vi "Gen_2D_Raster.vi"(0 "Fast-axis Para":T2={"Number of Steps"=100, "Max X"=5.0, "Min X"=-5.0}, 1 "Lissajous Cluster":cluster{"a":dbl, "b":dbl, "delta":dbl}={"a"=1.0, "b"=2.0, "delta"=0.0} {"delta" format="%_3g"; "b" format="%0.2p"; "a" format="%_3g"}, 2 "error in (no error)":errorcluster, 3 "Soften":bool, 4 "Pattern":T3(ring)=enum."Single Direction (Uniform)", 5 "Reset slow axis at End of Scan?":bool=TRUE, 8 "asymmetry":dbl=0.9, 9 "Soften points":i32=3, 10 "Slow-axis Para":T1={"Number of Steps"=10, "Max Y"=5.0, "Min Y"=-5.0}) -> (6 "2D Raster Pattern":dbl[][](graph)=[[0.0, 0.0, 0.0, 0.0, 0.0, 0.0, 0.0, 0.0, 0.0, 0.0, 0.5555555555555556, 0.5555555555555556, 0.5555555555555556, 0.5555555555555556, 0.5555555555555556, 0.5555555555555556, 0.5555555555555556, 0.5555555555555556, 0.5555555555555556, 0.5555555555555556, 1.1111111111111112, 1.1111111111111112, 1.1111111111111112, 1.1111111111111112, 1.1111111111111112, 1.1111111111111112, 1.1111111111111112, 1.1111111111111112, 1.1111111111111112, 1.1111111111111112, 1.6666666666666667, 1.6666666666666667, 1.6666666666666667, 1.6666666666666667, 1.6666666666666667, 1.6666666666666667, 1.6666666666666667, 1.6666666666666667, 1.6666666666666667, 1.6666666666666667, 2.2222222222222223, 2.2222222222222223, 2.2222222222222223, 2.2222222222222223, 2.2222222222222223, 2.2222222222222223, 2.2222222222222223, 2.2222222222222223, 2.2222222222222223, 2.2222222222222223, 2.7777777777777777, 2.7777777777777777, 2.7777777777777777, 2.7777777777777777, 2.7777777777777777, 2.7777777777777777, 2.7777777777777777, 2.7777777777777777, 2.7777777777777777, 2.7777777777777777, 3.3333333333333335, 3.3333333333333335, 3.3333333333333335, 3.3333333333333335, 3.3333333333333335, 3.3333333333333335, 3.3333333333333335, 3.3333333333333335, 3.3333333333333335, 3.3333333333333335, 3.8888888888888893, 3.8888888888888893, 3.8888888888888893, 3.8888888888888893, 3.8888888888888893, 3.8888888888888893, 3.8888888888888893, 3.8888888888888893, 3.8888888888888893, 3.8888888888888893, 4.444444444444445, 4.444444444444445, 4.444444444444445, 4.444444444444445, 4.444444444444445, 4.444444444444445, 4.444444444444445, 4.444444444444445, 4.444444444444445, 4.444444444444445, 5.0, 5.0, 5.0, 5.0, 5.0, 5.0, 5.0, 5.0, 5.0, 5.0, 5.0, 4.444444444444445, 3.8888888888888893, 3.3333333333333335, 2.7777777777777777, 2.2222222222222223, 1.6666666666666667, 1.1111111111111112, 0.5555555555555556, 0.0], [0.0, 0.5555555555555556, 1.1111111111111112, 1.6666666666666667, 2.2222222222222223, 2.7777777777777777, 3.3333333333333335, 3.8888888888888893, 4.444444444444445, 5.0, 5.0, 4.444444444444445, 3.8888888888888893, 3.3333333333333335, 2.7777777777777777, 2.2222222222222223, 1.6666666666666667, 1.1111111111111112, 0.5555555555555556, 0.0, 0.0, 0.5555555555555556, 1.1111111111111112, 1.6666666666666667, 2.2222222222222223, 2.7777777777777777, 3.3333333333333335, 3.8888888888888893, 4.444444444444445, 5.0, 5.0, 4.444444444444445, 3.8888888888888893, 3.3333333333333335, 2.7777777777777777, 2.2222222222222223, 1.6666666666666667, 1.1111111111111112, 0.5555555555555556, 0.0, 0.0, 0.5555555555555556, 1.1111111111111112, 1.6666666666666667, 2.2222222222222223, 2.7777777777777777, 3.3333333333333335, 3.8888888888888893, 4.444444444444445, 5.0, 5.0, 4.444444444444445, 3.8888888888888893, 3.3333333333333335, 2.7777777777777777, 2.2222222222222223, 1.6666666666666667, 1.1111111111111112, 0.5555555555555556, 0.0, 0.0, 0.5555555555555556, 1.1111111111111112, 1.6666666666666667, 2.2222222222222223, 2.7777777777777777, 3.3333333333333335, 3.8888888888888893, 4.444444444444445, 5.0, 5.0, 4.444444444444445, 3.8888888888888893, 3.3333333333333335, 2.7777777777777777, 2.2222222222222223, 1.6666666666666667, 1.1111111111111112, 0.5555555555555556, 0.0, 0.0, 0.5555555555555556, 1.1111111111111112, 1.6666666666666667, 2.2222222222222223, 2.7777777777777777, 3.3333333333333335, 3.8888888888888893, 4.444444444444445, 5.0, 5.0, 4.444444444444445, 3.8888888888888893, 3.3333333333333335, 2.7777777777777777, 2.2222222222222223, 1.6666666666666667, 1.1111111111111112, 0.5555555555555556, 0.0, 0.0, 0.0, 0.0, 0.0, 0.0, 0.0, 0.0, 0.0, 0.0, 0.0]], 7 "error IO":errorcluster)   [LabVIEW 2014]
uses:
  <vilib>/Analysis/1siggen.llb/Ramp Pattern by Samples.vi
  <vilib>/express/express arith-compare/Formula/XNode/ExpressFormulaBlockNode.xnode
  <vilib>/Analysis/NI_AALBase.lvlib
  <vilib>/gmath/NI_Gmath.lvlib
  <vilib>/measure/NI_MABase.lvlib
panel:
  out "2D  Pattern":dbl[][](graph)
  out "XY Graph 2":cluster{"Y":dbl[], "Y":dbl[]}[](graph) caption="XY Graph"
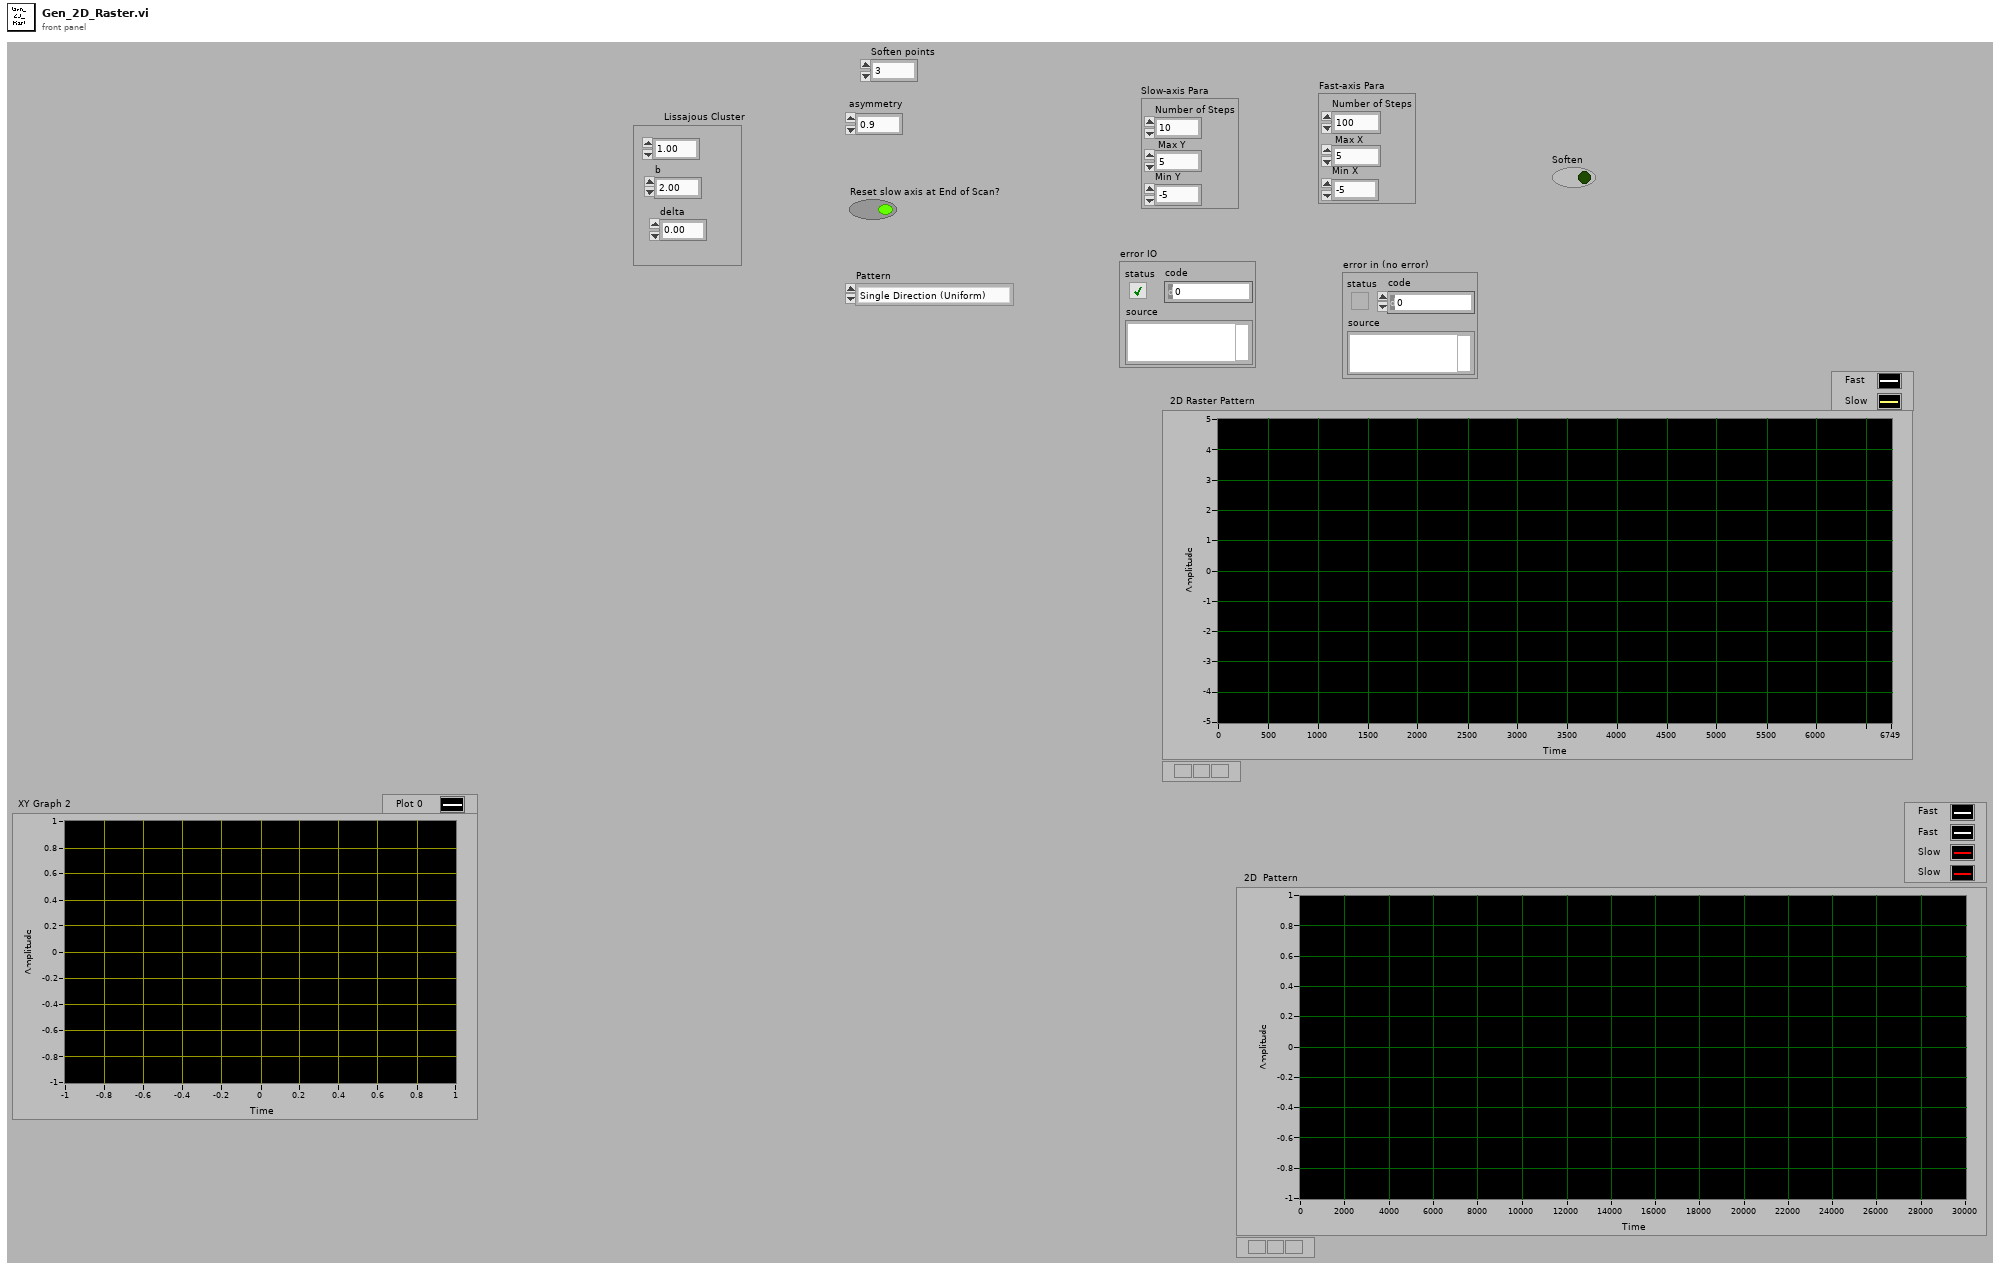
[diagram p1: front panel]
types:
  T1 = cluster{"Number of Steps":i32, "Max Y":dbl, "Min Y":dbl}
  T2 = cluster{"Number of Steps":i32, "Max X":dbl, "Min X":dbl}
  T3 = enum16{"Lissajous", "Adjustable sawtooth", "Single Direction (Uniform)", "Single Direction (Fast Reset)", "Bi-Directional"}
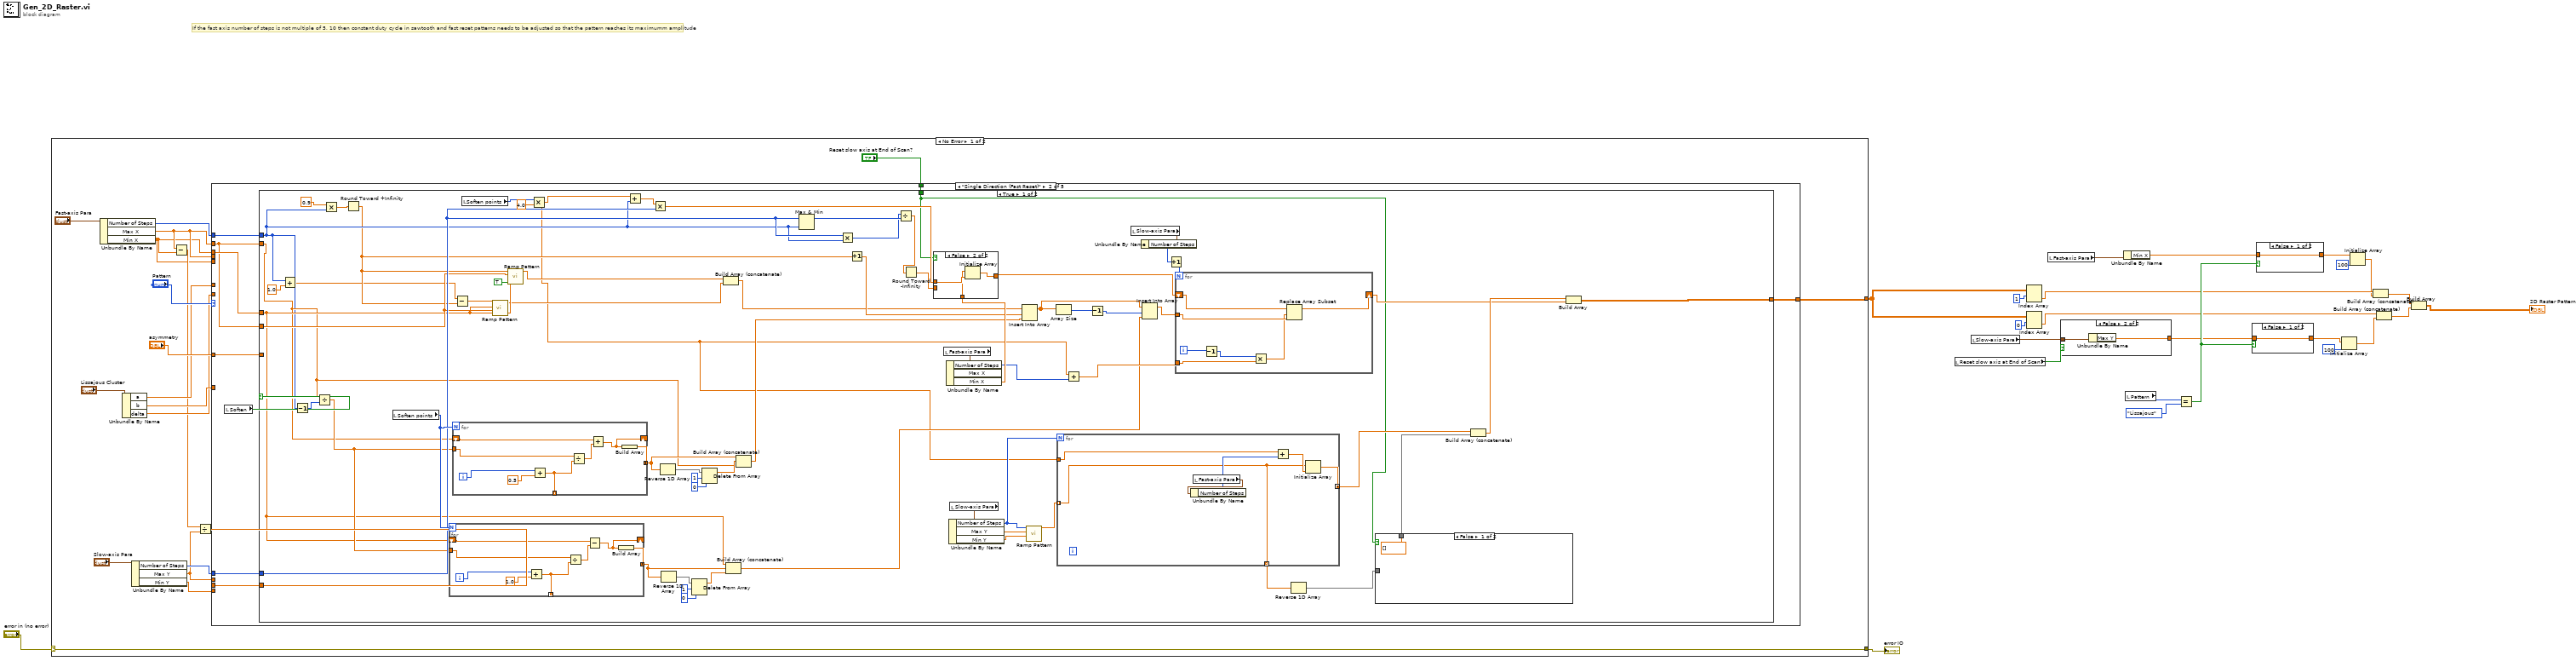
[diagram p0: block diagram]
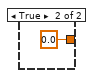
[diagram p2: hidden frame]
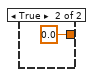
[diagram p3: hidden frame]
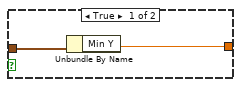
[diagram p4: hidden frame]
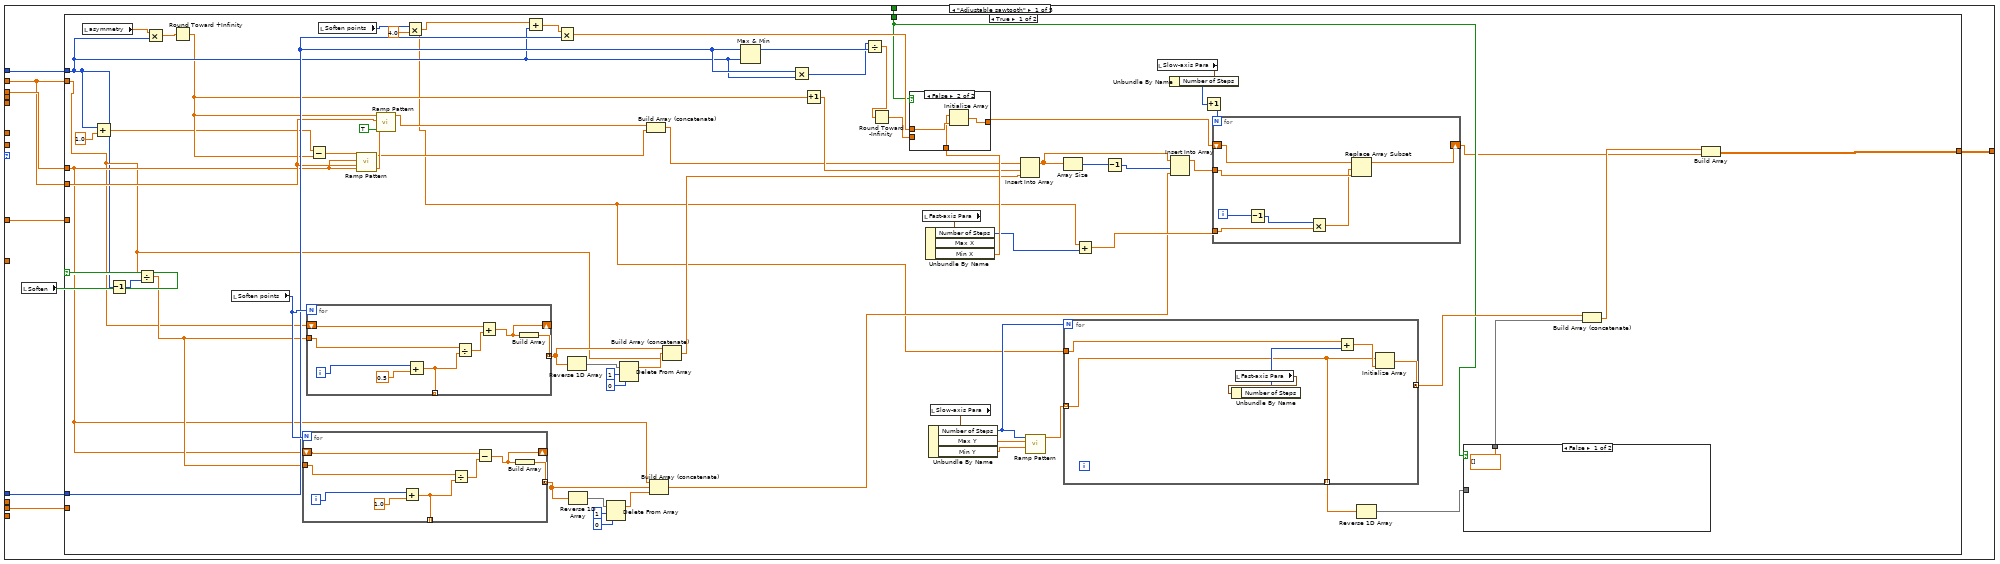
[diagram p5: hidden frame]
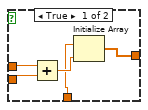
[diagram p7: hidden frame]
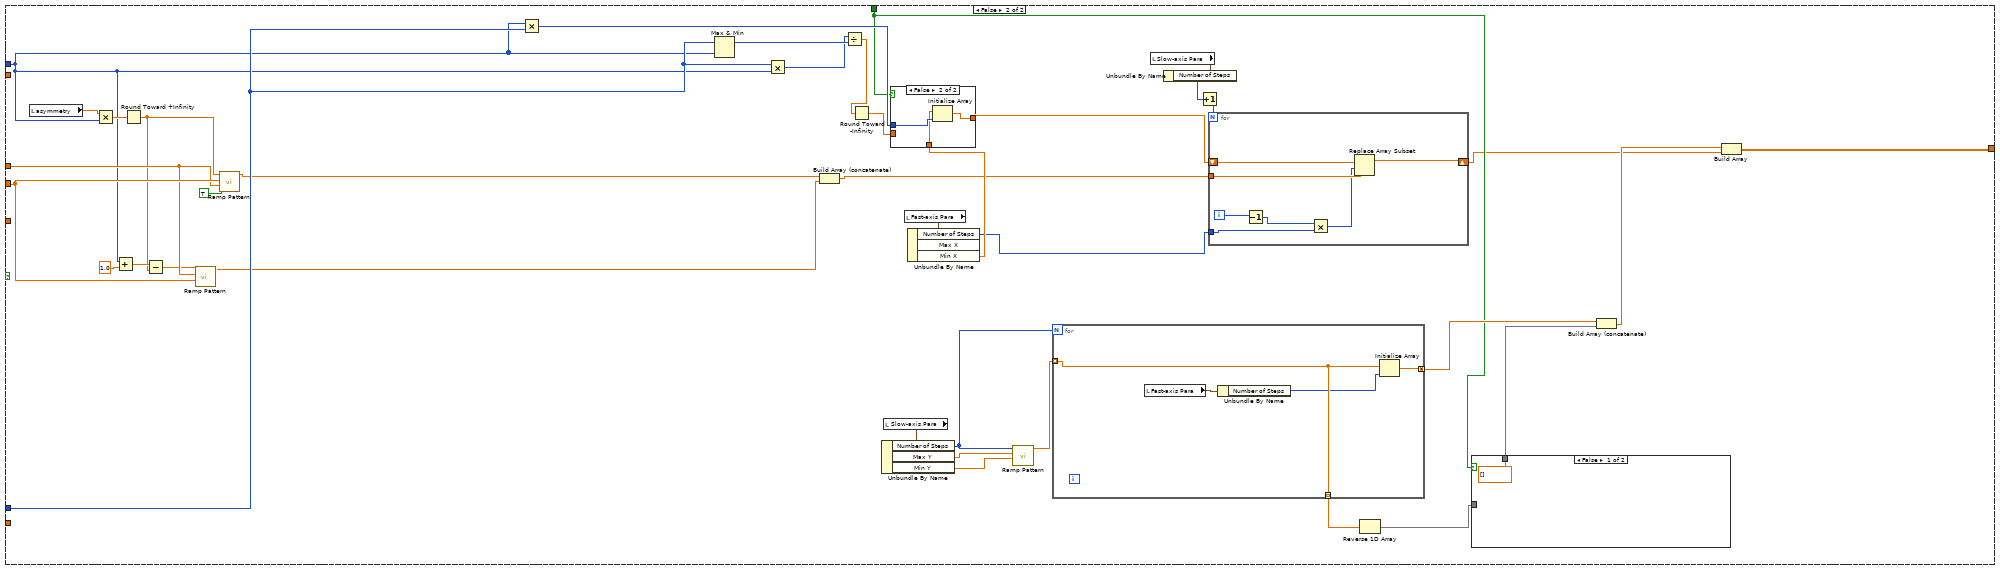
[diagram p8: hidden frame]
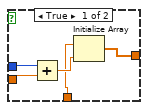
[diagram p10: hidden frame]
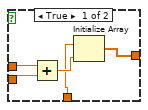
[diagram p12: hidden frame]
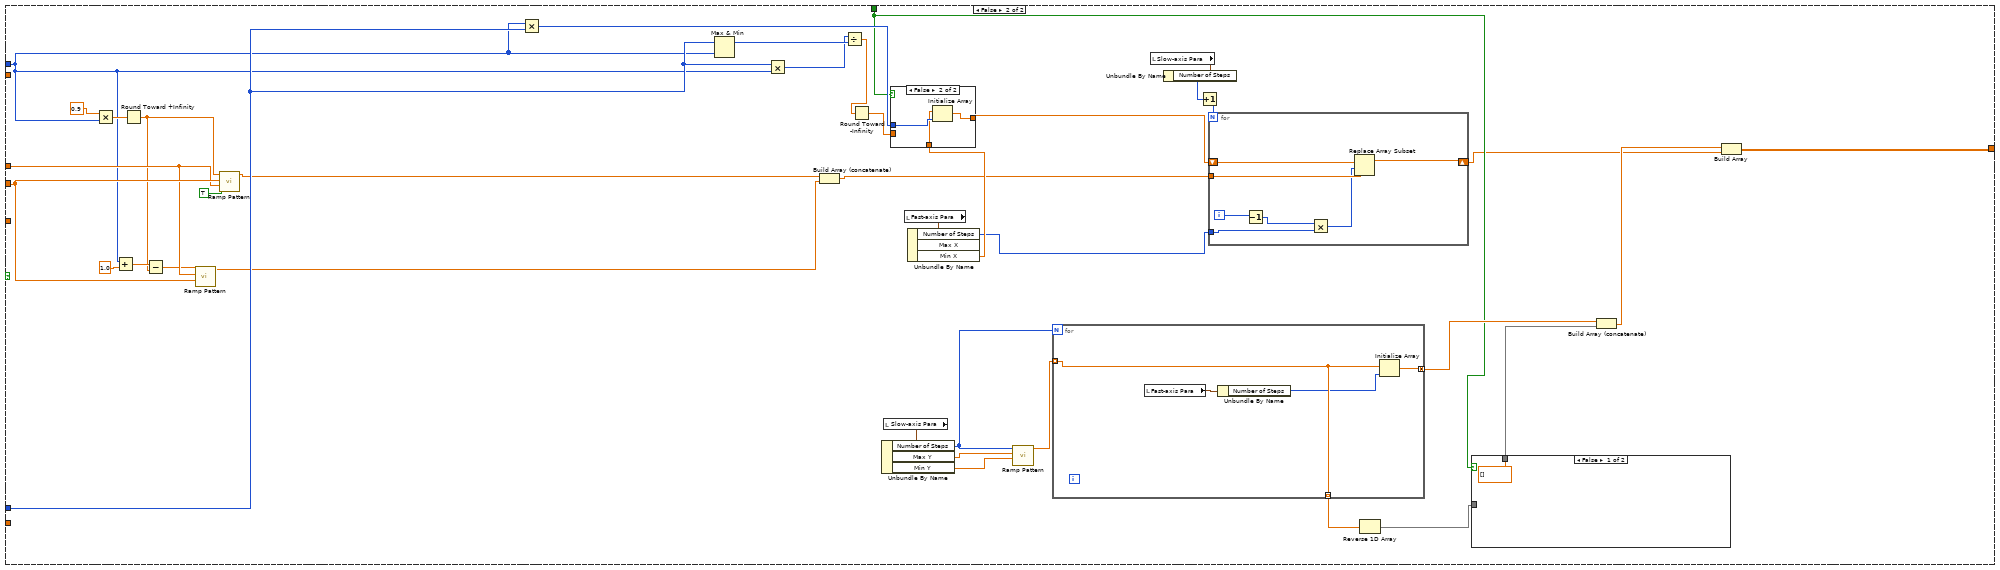
[diagram p13: hidden frame]
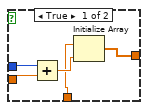
[diagram p15: hidden frame]
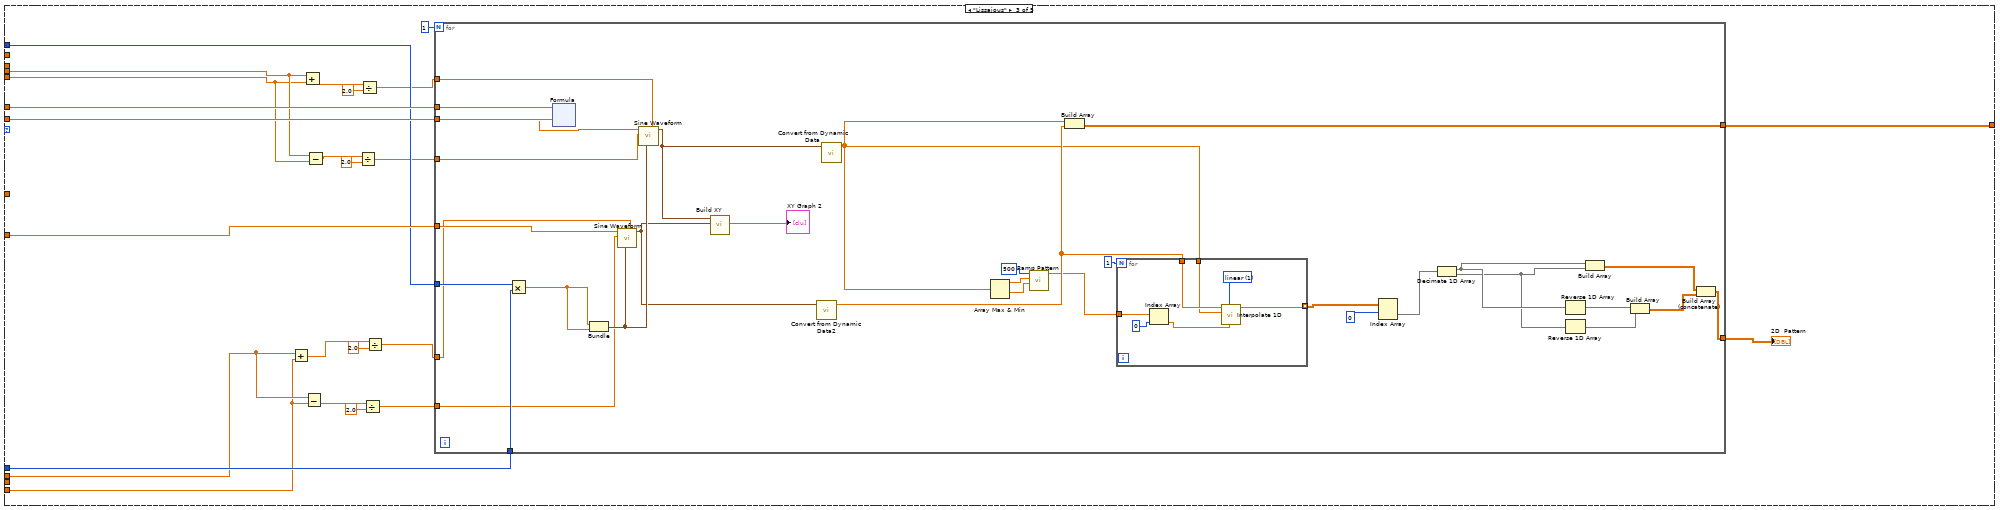
[diagram p16: hidden frame]
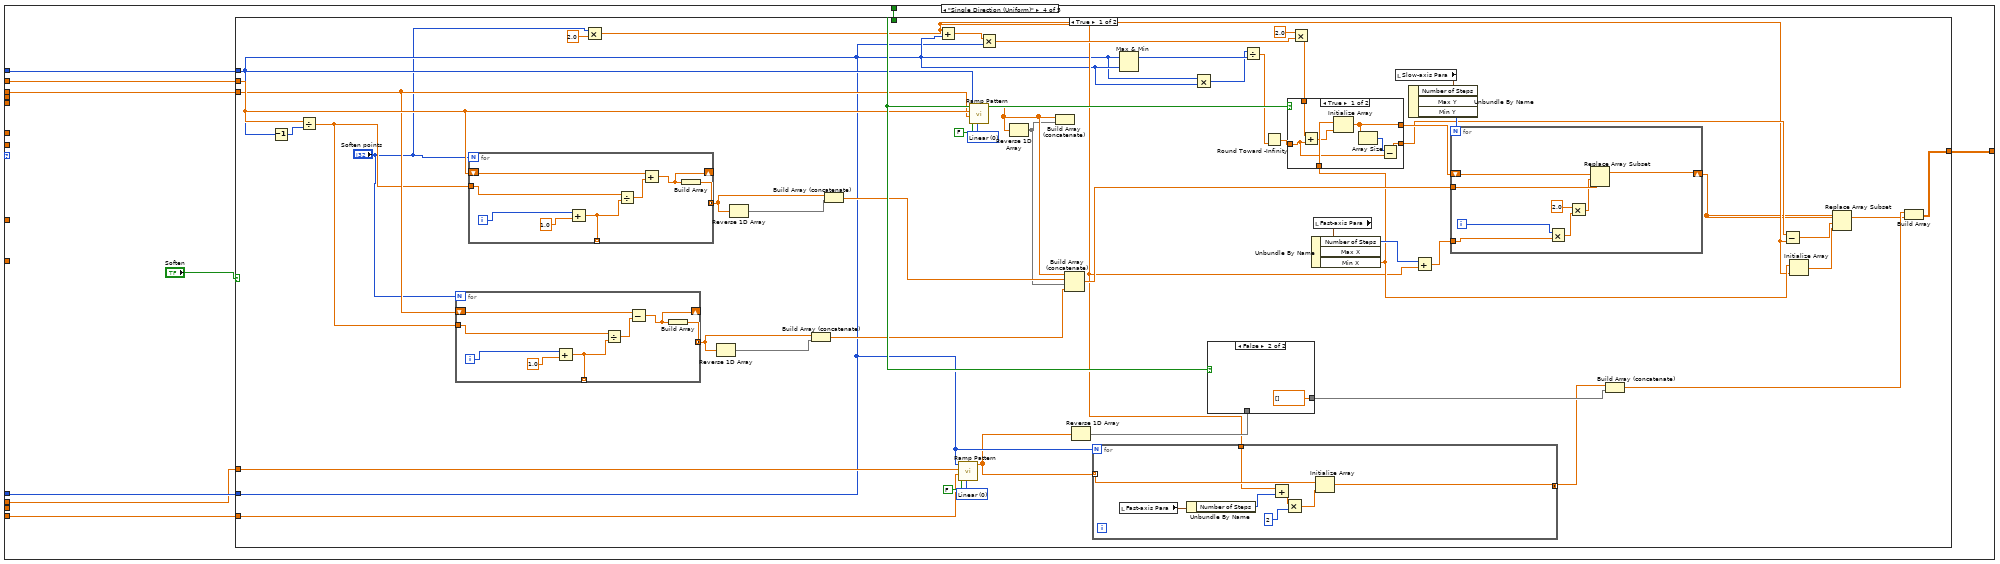
[diagram p17: hidden frame]
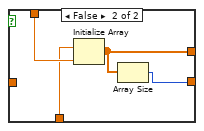
[diagram p19: hidden frame]
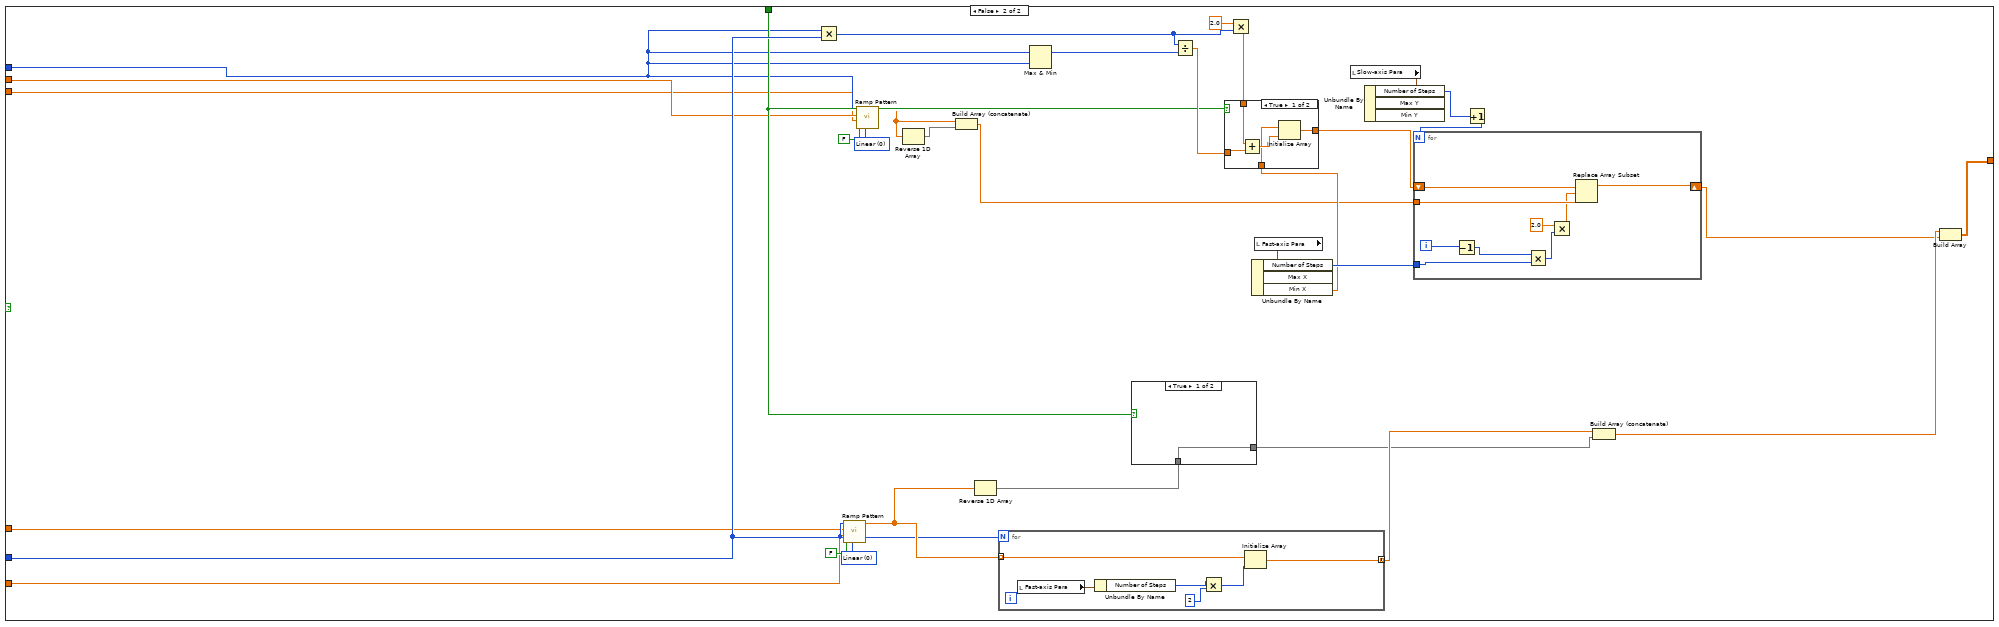
[diagram p20: hidden frame]
diagram:
  # "If the fast axis number of steps is not multiple of 5, 10 then constant duty cycle in sawtooth and fast reset patterns needs to be adjusted so that the pattern reaches its maximumm amplitude"
  n1 = case shown="No Error" "error in (no error)" {
    selector: "error in (no error)" -> [w38 w825]
    tunnel: [w38 w825] -> w21
    tunnel: [w25 dbl[][] []] -> w24
    frame No Error {
      n2 = Unbundle By Name("Fast-axis Para") -> ("Number of Steps"=w41:i32, "Max X"=w27:dbl, "Min X"=w26:dbl)
      n3 = Unbundle By Name("Lissajous Cluster") -> ("a"=w33:dbl, "b"=w34:dbl, "delta"=w32:dbl)
      n4 = Unbundle By Name("Slow-axis Para") -> ("Number of Steps"=w39:i32, "Max Y"=w31:dbl, "Min Y"=w28:dbl)
      n5 = Subtract(x=w27, y=w26) -> (x-y=w29:dbl)
      n6 = Divide(x=w29, y=w31) -> (x/y=w30:dbl)
      n7 = case shown="\"Single Direction (Fast Reset)\"" "Pattern" {
        tunnel: w41 -> [w49 w222 w410 w467 w634]
        tunnel: w27 -> [w44 w217 _ w466 w632]
        tunnel: w26 -> [w52 w225 _ w465 w631]
        tunnel: w30 -> [w51 w224 _ _ _]
        tunnel: w39 -> [w50 w223 w409 w472 w627]
        tunnel: "asymmetry" -> [w47 w220 _ _ _]
        tunnel: [w48 w221 w406 w470 w628] -> w25
        tunnel: "Reset slow axis at End of Scan?" -> [w46 w219 _ w471 w633]
        tunnel: w33 -> [_ _ w413 _ _]
        tunnel: w32 -> [_ _ w412 _ _]
        tunnel: w34 -> [_ _ w411 _ _]
        tunnel: w31 -> [_ _ w394 w469 w630]
        tunnel: w28 -> [_ _ w393 w468 w629]
        tunnel: w27 -> [_ _ w405 _ _]
        tunnel: w26 -> [_ _ w404 _ _]
        frame "Adjustable sawtooth" {
          n8 = local read "Soften"() -> (w45:bool)
          n9 = case shown="True" w45 {
            tunnel: w44 -> [w71 _]
            tunnel: w52 -> [w75 w173]
            tunnel: w51 -> [_ _]
            tunnel: w50 -> [w79 w176]
            tunnel: w49 -> [w69 w157]
            tunnel: [w111 w189] -> w48
            tunnel: w47 -> [_ _]
            tunnel: w46 -> [w82 w179]
            tunnel: w44 -> [w76 w174]
            frame True {
              n10 = local read "asymmetry"() -> (w74:dbl)
              n11 = Add(x=w69, y=1.0) -> (x+y=w59:dbl)
              n12 = Decrement(x=w69) -> (x-1=w99:i32)
              n13 = Divide(x=w71, y=w99) -> (x/y=w77:dbl)
              n14 = Multiply(x=w74, y=w69) -> (x*y=w73:dbl)
              n15 = Round Toward +Infinity(x=w73) -> (ceil(x): smallest int >= x=w60:dbl)
              n16 = local read "Soften points"() -> (w93:i32)
              n17 = for {
                N: w93 -> [_]
                tunnel: w77 -> [w123]
                tunnel: [w124] -> w98 mode=concatenating
                shift-right: [w121] -> _
                shift-left: w75 -> [w125]
                tunnel: [w118] -> _ mode=indexing
                i -> [w119]
                n18 = Add(x=w119, y=1.0) -> (x+y=w118:dbl)
                n19 = Divide(x=w123, y=w118) -> (x/y=w120:dbl)
                n20 = Subtract(x=w125, y=w120) -> (x-y=w121:dbl)
                n21 = Build Array(w121) -> (w124:dbl[])
              }
              n22 = for {
                N: w93 -> [_]
                tunnel: w77 -> [w131]
                tunnel: [w132] -> w103 mode=concatenating
                shift-right: [w129] -> _
                shift-left: w71 -> [w133]
                tunnel: [w126] -> _ mode=indexing
                i -> [w127]
                n23 = Add(x=w127, y=0.5) -> (x+y=w126:dbl)
                n24 = Divide(x=w131, y=w126) -> (x/y=w128:dbl)
                n25 = Add(x=w133, y=w128) -> (x+y=w129:dbl)
                n26 = Build Array(w129) -> (w132:dbl[])
              }
              n27 = Subtract(x=w59, y=w60) -> (x-y=w70:dbl)
              n28 = local read "Soften points"() -> (w88:i32)
              n29 = call-poly <vilib>:"Ramp Pattern.vi"("start"=w76, "end"=w75, "samples"=w70) -> ("Ramp Pattern"=w56:dbl[])  [unwired: 7 in, 1 out]
              n30 = call-poly <vilib>:"Ramp Pattern.vi"("exclude end?"=TRUE, "start"=w75, "end"=w76, "samples"=w60) -> ("Ramp Pattern"=w58:dbl[])  [unwired: 6 in, 1 out]
              n31 = Multiply(x=w88, y=4.0) -> (x*y=w54:dbl)
              n32 = Add(x=w54, y=w69) -> (x+y=w87:dbl)
              n33 = Multiply(x=w87, y=w79) -> (x*y=w116:dbl)
              n34 = Reverse 1D Array(array=w103) -> (reversed array=w102:dbl[])
              n35 = Reverse 1D Array(array=w98) -> (reversed array=w97:dbl[])
              n36 = Delete From Array(array=w97, length=1, index=0) -> (array with subset deleted=w94:dbl[])  [unwired: 1 out]
              n37 = Delete From Array(array=w102, length=1, index=0) -> (array with subset deleted=w91:dbl[])  [unwired: 1 out]
              n38 = Build Array (concatenate)(w58, w56) -> (w67:dbl[])
              n39 = Build Array (concatenate)(w75, w98, w94) -> (w55:dbl[])
              n40 = Build Array (concatenate)(w103, w91, w71) -> (w57:dbl[])
              n41 = Max & Min(x=w79, y=w69) -> (max(x,y)=w115:i32)  [unwired: 1 out]
              n42 = Multiply(x=w79, y=w69) -> (x*y=w78:i32)
              n43 = Increment(x=w60) -> (x+1=w92:dbl)
              n44 = Divide(x=w78, y=w115) -> (x/y=w86:dbl)
              n45 = Round Toward -Infinity(1:w86) -> (0:w85:dbl)
              n46 = local read "Fast-axis Para"() -> (w114:T2)
              n47 = Unbundle By Name(w114) -> ("Number of Steps"=w84:i32, "Min X"=w108:dbl)  [unwired: 1 out]
              n48 = case shown="False" w82 {
                tunnel: [w140 w143] -> w117
                tunnel: w116 -> [w139 w142]
                tunnel: w85 -> [w138 _]
                tunnel: w108 -> [w136 w141]
                frame True {
                  n49 = Add(x=w139, y=w138) -> (x+y=w137:dbl)
                  n50 = Initialize Array(w136, w137) -> (w140:dbl[])
                }
                frame False {
                  n51 = Initialize Array(w141, w142) -> (w143:dbl[])
                }
              }
              n52 = local read "Slow-axis Para"() -> (w112:T1)
              n53 = Unbundle By Name(w112) -> ("Number of Steps"=w64:i32, "Max Y"=w63:dbl, "Min Y"=w62:dbl)
              n54 = Insert Into Array(array=w67, index=w92, new element=w57) -> (w90:dbl[])
              n55 = call-poly <vilib>:"Ramp Pattern.vi"("start"=w62, "end"=w63, "samples"=w64) -> ("Ramp Pattern"=w61:dbl[])  [unwired: 7 in, 1 out]
              n56 = Array Size(array=w90) -> (size(s)=w66:i32)
              n57 = for {
                N: w64 -> [_]
                tunnel: w61 -> [w144] mode=indexing
                tunnel: [w148] -> w104 mode=concatenating
                tunnel: [w144] -> w106 mode=indexing
                tunnel: w54 -> [w147]
                n58 = local read "Fast-axis Para"() -> (w149:T2)
                n59 = Unbundle By Name(w149) -> ("Number of Steps"=w146:i32)
                n60 = Add(x=w147, y=w146) -> (x+y=w145:dbl)
                n61 = Initialize Array(w144, w145) -> (w148:dbl[])
              }
              n62 = Add(x=w54, y=w84) -> (x+y=w83:dbl)
              n63 = Decrement(x=w66) -> (x-1=w65:i32)
              n64 = local read "Slow-axis Para"() -> (w113:T1)
              n65 = Unbundle By Name(w113) -> ("Number of Steps"=w110:i32)
              n66 = Insert Into Array(array=w90, index=w65, new element=w55) -> (w53:dbl[])
              n67 = Increment(x=w110) -> (x+1=w109:i32)
              n68 = for {
                N: w109 -> [_]
                tunnel: w53 -> [w156]
                shift-right: [w154] -> w80
                shift-left: w117 -> [w155]
                tunnel: w83 -> [w152]
                i -> [w151]
                n69 = Decrement(x=w151) -> (x-1=w150:i32)
                n70 = Multiply(x=w150, y=w152) -> (x*y=w153:dbl)
                n71 = Replace Array Subset(array=w155, new element=w156, index=w153) -> (w154:dbl[])
              }
              n72 = Reverse 1D Array(array=w106) -> (reversed array=w105:dbl[])
              n73 = case shown="False" w82 {
                tunnel: w105 -> [_ w135]
                tunnel: [dbl[] [] w135] -> w107
                frame False {
                }
                frame True {
                }
              }
              n74 = Build Array (concatenate)(w104, w107) -> (w81:dbl[])
              n75 = Build Array(w81, w80) -> (w111:dbl[][])
            }
            frame False {
              n76 = local read "asymmetry"() -> (w172:dbl)
              n77 = Multiply(x=w172, y=w157) -> (x*y=w171:dbl)
              n78 = Add(x=w157, y=1.0) -> (x+y=w169:dbl)
              n79 = Round Toward +Infinity(x=w171) -> (ceil(x): smallest int >= x=w160:dbl)
              n80 = Subtract(x=w169, y=w160) -> (x-y=w168:dbl)
              n81 = call-poly <vilib>:"Ramp Pattern.vi"("start"=w174, "end"=w173, "samples"=w168) -> ("Ramp Pattern"=w166:dbl[])  [unwired: 7 in, 1 out]
              n82 = call-poly <vilib>:"Ramp Pattern.vi"("exclude end?"=TRUE, "start"=w173, "end"=w174, "samples"=w160) -> ("Ramp Pattern"=w165:dbl[])  [unwired: 6 in, 1 out]
              n83 = Multiply(x=w157, y=w176) -> (x*y=w194:i32)
              n84 = Max & Min(x=w176, y=w157) -> (max(x,y)=w193:i32)  [unwired: 1 out]
              n85 = Multiply(x=w176, y=w157) -> (x*y=w175:i32)
              n86 = Build Array (concatenate)(w165, w166) -> (w159:dbl[])
              n87 = Divide(x=w175, y=w193) -> (x/y=w181:dbl)
              n88 = Round Toward -Infinity(1:w181) -> (0:w180:dbl)
              n89 = local read "Slow-axis Para"() -> (w190:T1)
              n90 = Unbundle By Name(w190) -> ("Number of Steps"=w164:i32, "Max Y"=w163:dbl, "Min Y"=w162:dbl)
              n91 = local read "Fast-axis Para"() -> (w192:T2)
              n92 = Unbundle By Name(w192) -> ("Number of Steps"=w158:i32, "Min X"=w186:dbl)  [unwired: 1 out]
              n93 = case shown="False" w179 {
                tunnel: [w202 w205] -> w195
                tunnel: w194 -> [w201 w204]
                tunnel: w180 -> [w200 _]
                tunnel: w186 -> [w198 w203]
                frame True {
                  n94 = Add(x=w201, y=w200) -> (x+y=w199:dbl)
                  n95 = Initialize Array(w198, w199) -> (w202:dbl[])
                }
                frame False {
                  n96 = Initialize Array(w203, w204) -> (w205:dbl[])
                }
              }
              n97 = call-poly <vilib>:"Ramp Pattern.vi"("start"=w162, "end"=w163, "samples"=w164) -> ("Ramp Pattern"=w161:dbl[])  [unwired: 7 in, 1 out]
              n98 = for {
                N: w164 -> [_]
                tunnel: w161 -> [w207] mode=indexing
                tunnel: [w208] -> w182 mode=concatenating
                tunnel: [w207] -> w184 mode=indexing
                n99 = local read "Fast-axis Para"() -> (w209:T2)
                n100 = Unbundle By Name(w209) -> ("Number of Steps"=w206:i32)
                n101 = Initialize Array(w207, w206) -> (w208:dbl[])
              }
              n102 = local read "Slow-axis Para"() -> (w191:T1)
              n103 = Unbundle By Name(w191) -> ("Number of Steps"=w188:i32)
              n104 = Increment(x=w188) -> (x+1=w187:i32)
              n105 = for {
                N: w187 -> [_]
                tunnel: w159 -> [w216]
                shift-right: [w214] -> w177
                shift-left: w195 -> [w215]
                tunnel: w158 -> [w212]
                i -> [w211]
                n106 = Decrement(x=w211) -> (x-1=w210:i32)
                n107 = Multiply(x=w210, y=w212) -> (x*y=w213:i32)
                n108 = Replace Array Subset(array=w215, new element=w216, index=w213) -> (w214:dbl[])
              }
              n109 = Reverse 1D Array(array=w184) -> (reversed array=w183:dbl[])
              n110 = case shown="False" w179 {
                tunnel: w183 -> [_ w197]
                tunnel: [dbl[] [] w197] -> w185
                frame False {
                }
                frame True {
                }
              }
              n111 = Build Array (concatenate)(w182, w185) -> (w178:dbl[])
              n112 = Build Array(w178, w177) -> (w189:dbl[][])
            }
          }
        }
        frame "Single Direction (Fast Reset)" {
          n113 = local read "Soften"() -> (w218:bool)
          n114 = case shown="True" w218 {
            tunnel: w217 -> [w246 _]
            tunnel: w225 -> [w249 w346]
            tunnel: w224 -> [_ _]
            tunnel: w223 -> [w253 w349]
            tunnel: w222 -> [w244 w331]
            tunnel: [w284 w362] -> w221
            tunnel: w220 -> [_ _]
            tunnel: w219 -> [w226 w352]
            tunnel: w217 -> [w250 w347]
            frame True {
              n115 = Add(x=w244, y=1.0) -> (x+y=w234:dbl)
              n116 = Decrement(x=w244) -> (x-1=w272:i32)
              n117 = Divide(x=w246, y=w272) -> (x/y=w251:dbl)
              n118 = Multiply(x=0.9 ("asymmetry"), y=w244) -> (x*y=w248:dbl)
              n119 = Round Toward +Infinity(x=w248) -> (ceil(x): smallest int >= x=w235:dbl)
              n120 = local read "Soften points"() -> (w266:i32)
              n121 = for {
                N: w266 -> [_]
                tunnel: w251 -> [w296]
                tunnel: [w297] -> w271 mode=concatenating
                shift-right: [w294] -> _
                shift-left: w249 -> [w298]
                tunnel: [w291] -> _ mode=indexing
                i -> [w292]
                n122 = Add(x=w292, y=1.0) -> (x+y=w291:dbl)
                n123 = Divide(x=w296, y=w291) -> (x/y=w293:dbl)
                n124 = Subtract(x=w298, y=w293) -> (x-y=w294:dbl)
                n125 = Build Array(w294) -> (w297:dbl[])
              }
              n126 = for {
                N: w266 -> [_]
                tunnel: w251 -> [w304]
                tunnel: [w305] -> w276 mode=concatenating
                shift-right: [w302] -> _
                shift-left: w246 -> [w306]
                tunnel: [w299] -> _ mode=indexing
                i -> [w300]
                n127 = Add(x=w300, y=0.5) -> (x+y=w299:dbl)
                n128 = Divide(x=w304, y=w299) -> (x/y=w301:dbl)
                n129 = Add(x=w306, y=w301) -> (x+y=w302:dbl)
                n130 = Build Array(w302) -> (w305:dbl[])
              }
              n131 = Subtract(x=w234, y=w235) -> (x-y=w245:dbl)
              n132 = local read "Soften points"() -> (w261:i32)
              n133 = call-poly <vilib>:"Ramp Pattern.vi"("start"=w250, "end"=w249, "samples"=w245) -> ("Ramp Pattern"=w231:dbl[])  [unwired: 7 in, 1 out]
              n134 = call-poly <vilib>:"Ramp Pattern.vi"("exclude end?"=TRUE, "start"=w249, "end"=w250, "samples"=w235) -> ("Ramp Pattern"=w233:dbl[])  [unwired: 6 in, 1 out]
              n135 = Multiply(x=w261, y=4.0) -> (x*y=w229:dbl)
              n136 = Add(x=w229, y=w244) -> (x+y=w260:dbl)
              n137 = Multiply(x=w260, y=w253) -> (x*y=w289:dbl)
              n138 = Reverse 1D Array(array=w276) -> (reversed array=w275:dbl[])
              n139 = Reverse 1D Array(array=w271) -> (reversed array=w270:dbl[])
              n140 = Delete From Array(array=w270, length=1, index=0) -> (array with subset deleted=w267:dbl[])  [unwired: 1 out]
              n141 = Delete From Array(array=w275, length=1, index=0) -> (array with subset deleted=w264:dbl[])  [unwired: 1 out]
              n142 = Build Array (concatenate)(w233, w231) -> (w242:dbl[])
              n143 = Build Array (concatenate)(w249, w271, w267) -> (w230:dbl[])
              n144 = Build Array (concatenate)(w276, w264, w246) -> (w232:dbl[])
              n145 = Max & Min(x=w253, y=w244) -> (max(x,y)=w288:i32)  [unwired: 1 out]
              n146 = Multiply(x=w253, y=w244) -> (x*y=w252:i32)
              n147 = Increment(x=w235) -> (x+1=w265:dbl)
              n148 = Divide(x=w252, y=w288) -> (x/y=w259:dbl)
              n149 = Round Toward -Infinity(1:w259) -> (0:w258:dbl)
              n150 = local read "Fast-axis Para"() -> (w287:T2)
              n151 = Unbundle By Name(w287) -> ("Number of Steps"=w257:i32, "Min X"=w281:dbl)  [unwired: 1 out]
              n152 = case shown="False" w226 {
                tunnel: [w313 w316] -> w290
                tunnel: w289 -> [w312 w315]
                tunnel: w258 -> [w311 _]
                tunnel: w281 -> [w309 w314]
                frame True {
                  n153 = Add(x=w312, y=w311) -> (x+y=w310:dbl)
                  n154 = Initialize Array(w309, w310) -> (w313:dbl[])
                }
                frame False {
                  n155 = Initialize Array(w314, w315) -> (w316:dbl[])
                }
              }
              n156 = local read "Slow-axis Para"() -> (w285:T1)
              n157 = Unbundle By Name(w285) -> ("Number of Steps"=w239:i32, "Max Y"=w238:dbl, "Min Y"=w237:dbl)
              n158 = Insert Into Array(array=w242, index=w265, new element=w232) -> (w263:dbl[])
              n159 = call-poly <vilib>:"Ramp Pattern.vi"("start"=w237, "end"=w238, "samples"=w239) -> ("Ramp Pattern"=w236:dbl[])  [unwired: 7 in, 1 out]
              n160 = Array Size(array=w263) -> (size(s)=w241:i32)
              n161 = for {
                N: w239 -> [_]
                tunnel: w236 -> [w317] mode=indexing
                tunnel: [w321] -> w277 mode=concatenating
                tunnel: [w317] -> w279 mode=indexing
                tunnel: w229 -> [w320]
                n162 = local read "Fast-axis Para"() -> (w322:T2)
                n163 = Unbundle By Name(w322) -> ("Number of Steps"=w319:i32)
                n164 = Add(x=w320, y=w319) -> (x+y=w318:dbl)
                n165 = Initialize Array(w317, w318) -> (w321:dbl[])
              }
              n166 = Add(x=w229, y=w257) -> (x+y=w256:dbl)
              n167 = Decrement(x=w241) -> (x-1=w240:i32)
              n168 = local read "Slow-axis Para"() -> (w286:T1)
              n169 = Unbundle By Name(w286) -> ("Number of Steps"=w283:i32)
              n170 = Insert Into Array(array=w263, index=w240, new element=w230) -> (w228:dbl[])
              n171 = Increment(x=w283) -> (x+1=w282:i32)
              n172 = for {
                N: w282 -> [_]
                tunnel: w228 -> [w329]
                shift-right: [w327] -> w254
                shift-left: w290 -> [w328]
                tunnel: w256 -> [w325]
                i -> [w324]
                n173 = Decrement(x=w324) -> (x-1=w323:i32)
                n174 = Multiply(x=w323, y=w325) -> (x*y=w326:dbl)
                n175 = Replace Array Subset(array=w328, new element=w329, index=w326) -> (w327:dbl[])
              }
              n176 = Reverse 1D Array(array=w279) -> (reversed array=w278:dbl[])
              n177 = case shown="False" w226 {
                tunnel: w278 -> [_ w308]
                tunnel: [dbl[] [] w308] -> w280
                frame False {
                }
                frame True {
                }
              }
              n178 = Build Array (concatenate)(w277, w280) -> (w255:dbl[])
              n179 = Build Array(w255, w254) -> (w284:dbl[][])
            }
            frame False {
              n180 = Multiply(x=0.9 ("asymmetry"), y=w331) -> (x*y=w345:dbl)
              n181 = Add(x=w331, y=1.0) -> (x+y=w343:dbl)
              n182 = Round Toward +Infinity(x=w345) -> (ceil(x): smallest int >= x=w334:dbl)
              n183 = Subtract(x=w343, y=w334) -> (x-y=w342:dbl)
              n184 = call-poly <vilib>:"Ramp Pattern.vi"("start"=w347, "end"=w346, "samples"=w342) -> ("Ramp Pattern"=w340:dbl[])  [unwired: 7 in, 1 out]
              n185 = call-poly <vilib>:"Ramp Pattern.vi"("exclude end?"=TRUE, "start"=w346, "end"=w347, "samples"=w334) -> ("Ramp Pattern"=w339:dbl[])  [unwired: 6 in, 1 out]
              n186 = Multiply(x=w331, y=w349) -> (x*y=w367:i32)
              n187 = Max & Min(x=w349, y=w331) -> (max(x,y)=w366:i32)  [unwired: 1 out]
              n188 = Multiply(x=w349, y=w331) -> (x*y=w348:i32)
              n189 = Build Array (concatenate)(w339, w340) -> (w333:dbl[])
              n190 = Divide(x=w348, y=w366) -> (x/y=w354:dbl)
              n191 = Round Toward -Infinity(1:w354) -> (0:w353:dbl)
              n192 = local read "Slow-axis Para"() -> (w363:T1)
              n193 = Unbundle By Name(w363) -> ("Number of Steps"=w338:i32, "Max Y"=w337:dbl, "Min Y"=w336:dbl)
              n194 = local read "Fast-axis Para"() -> (w365:T2)
              n195 = Unbundle By Name(w365) -> ("Number of Steps"=w332:i32, "Min X"=w359:dbl)  [unwired: 1 out]
              n196 = case shown="False" w352 {
                tunnel: [w375 w378] -> w368
                tunnel: w367 -> [w374 w377]
                tunnel: w353 -> [w373 _]
                tunnel: w359 -> [w371 w376]
                frame True {
                  n197 = Add(x=w374, y=w373) -> (x+y=w372:dbl)
                  n198 = Initialize Array(w371, w372) -> (w375:dbl[])
                }
                frame False {
                  n199 = Initialize Array(w376, w377) -> (w378:dbl[])
                }
              }
              n200 = call-poly <vilib>:"Ramp Pattern.vi"("start"=w336, "end"=w337, "samples"=w338) -> ("Ramp Pattern"=w335:dbl[])  [unwired: 7 in, 1 out]
              n201 = for {
                N: w338 -> [_]
                tunnel: w335 -> [w380] mode=indexing
                tunnel: [w381] -> w355 mode=concatenating
                tunnel: [w380] -> w357 mode=indexing
                n202 = local read "Fast-axis Para"() -> (w382:T2)
                n203 = Unbundle By Name(w382) -> ("Number of Steps"=w379:i32)
                n204 = Initialize Array(w380, w379) -> (w381:dbl[])
              }
              n205 = local read "Slow-axis Para"() -> (w364:T1)
              n206 = Unbundle By Name(w364) -> ("Number of Steps"=w361:i32)
              n207 = Increment(x=w361) -> (x+1=w360:i32)
              n208 = for {
                N: w360 -> [_]
                tunnel: w333 -> [w389]
                shift-right: [w387] -> w350
                shift-left: w368 -> [w388]
                tunnel: w332 -> [w385]
                i -> [w384]
                n209 = Decrement(x=w384) -> (x-1=w383:i32)
                n210 = Multiply(x=w383, y=w385) -> (x*y=w386:i32)
                n211 = Replace Array Subset(array=w388, new element=w389, index=w386) -> (w387:dbl[])
              }
              n212 = Reverse 1D Array(array=w357) -> (reversed array=w356:dbl[])
              n213 = case shown="False" w352 {
                tunnel: w356 -> [_ w370]
                tunnel: [dbl[] [] w370] -> w358
                frame False {
                }
                frame True {
                }
              }
              n214 = Build Array (concatenate)(w355, w358) -> (w351:dbl[])
              n215 = Build Array(w351, w350) -> (w362:dbl[][])
            }
          }
        }
        frame "Lissajous" {
          n216 = Add(x=w394, y=w393) -> (x+y=w396:dbl)
          n217 = Add(x=w405, y=w404) -> (x+y=w399:dbl)
          n218 = Subtract(x=w394, y=w393) -> (x-y=w391:dbl)
          n219 = Subtract(x=w405, y=w404) -> (x-y=w402:dbl)
          n220 = Divide(x=w402, y=2.0) -> (x/y=w401:dbl)
          n221 = Divide(x=w399, y=2.0) -> (x/y=w398:dbl)
          n222 = Divide(x=w391, y=2.0) -> (x/y=w390:dbl)
          n223 = Divide(x=w396, y=2.0) -> (x/y=w395:dbl)
          n224 = for {
            N: 1 -> [_]
            tunnel: w413 -> [w446]
            tunnel: w412 -> [w445]
            tunnel: w411 -> [w444]
            tunnel: w410 -> [w443]
            tunnel: w409 -> [w442]
            tunnel: [w441] -> w406
            tunnel: [w419] -> w407
            tunnel: w398 -> [w418]
            tunnel: w395 -> [w417]
            tunnel: w401 -> [w416]
            tunnel: w390 -> [w415]
            n225 = Multiply(x=w443, y=w442) -> (x*y=w414:dbl)
            n226 = xnode "Formula"("a"=w446, "delta"=w445) -> ("Result"=w440:dbl)  [unwired: 1 in, 1 out]
            n227 = Bundle(w414, w414) -> (w439:cluster{dbl, dbl})  [unwired: 1 in]
            n228 = call <vilib>:"Sine Waveform.vi"("offset"=w417, "sampling info"=w439, "amplitude"=w415, "frequency"=w444) -> ("signal out"=w434:waveform(dbl))  [unwired: 6 in, 1 out]
            n229 = call <vilib>:"Sine Waveform.vi"("offset"=w418, "sampling info"=w439, "amplitude"=w416, "frequency"=w440) -> ("signal out"=w435:waveform(dbl))  [unwired: 6 in, 1 out]
            n230 = call "Build XY"("Y Input"=w434, "X Input"=w435) -> ("XY Graph"=→"XY Graph 2":cluster{"Y":dbl[], "Y":dbl[]}[])  [unwired: 3 in, 6 out]
            n231 = call "Convert from Dynamic Data2"("Dynamic Data Type"=w434) -> ("Array"=w437:dbl[])  [unwired: 3 in]
            n232 = call "Convert from Dynamic Data"("Dynamic Data Type"=w435) -> ("Array"=w436:dbl[])  [unwired: 3 in]
            n233 = Array Max & Min(array=w436) -> (max value=w433:dbl, min value=w432:dbl)  [unwired: 2 out]
            n234 = call-poly <vilib>:"Ramp Pattern.vi"("start"=w432, "end"=w433, "samples"=500 ("# of Samples")) -> ("Ramp Pattern"=w429:dbl[])  [unwired: 7 in, 1 out]
            n235 = Build Array(w436, w437) -> (w441:dbl[][])
            n236 = for {
              N: 1 -> [_]
              tunnel: w437 -> [w453]
              tunnel: w436 -> [w452]
              tunnel: w429 -> [w450]
              tunnel: [w447] -> w427 mode=indexing
              w449 = 1 items=["nearest", "linear", "spline", "cubic Hermite", "Lagrange"] ("method")
              n237 = Index Array(array=w450, index=0) -> (element=w451:dbl)
              n238 = call <vilib>:"Interpolate 1D.vi"("ntimes"=w451, "method"=w449, "X"=w452, "Y"=w453) -> ("yi"=w447:dbl[])  [unwired: 5 in, 2 out]
            }
            n239 = Index Array(array=w427, index (row)=u8 0) -> (element=w420:dbl[])  [unwired: 1 in]
            n240 = Decimate 1D Array(w420) -> (w426:dbl[], w425:dbl[])
            n241 = Reverse 1D Array(array=w426) -> (reversed array=w424:dbl[])
            n242 = Reverse 1D Array(array=w425) -> (reversed array=w423:dbl[])
            n243 = Build Array(w426, w425) -> (w422:dbl[][])
            n244 = Build Array(w424, w423) -> (w421:dbl[][])
            n245 = Build Array (concatenate)(w422, w421) -> (w419:dbl[][])
          }
          "2D  Pattern" <- w407
        }
        frame "Single Direction (Uniform)" {
          n246 = case shown="True" "Soften" {
            tunnel: w472 -> [w478 w579]
            tunnel: w471 -> [w510 w578]
            tunnel: [w509 w577] -> w470
            tunnel: w469 -> [w508 w576]
            tunnel: w468 -> [w507 w575]
            tunnel: w467 -> [w479 w572]
            tunnel: w466 -> [w506 w571]
            tunnel: w465 -> [w499 w570]
            frame True {
              w514 = u16 0 items=["Linear", "Logarithmic"] ("type")
              w516 = u16 0 items=["Linear", "Logarithmic"] ("type")
              n247 = Decrement(x=w479) -> (x-1=w501:i32)
              n248 = Divide(x=w506, y=w501) -> (x/y=w498:dbl)
              n249 = for {
                N: "Soften points" -> [_]
                tunnel: w498 -> [w528]
                tunnel: [w529] -> w500 mode=concatenating
                shift-right: [w526] -> _
                shift-left: w499 -> [w530]
                tunnel: [w523] -> _ mode=indexing
                i -> [w524]
                n250 = Add(x=w524, y=1.0) -> (x+y=w523:dbl)
                n251 = Divide(x=w528, y=w523) -> (x/y=w525:dbl)
                n252 = Subtract(x=w530, y=w525) -> (x-y=w526:dbl)
                n253 = Build Array(w526) -> (w529:dbl[])
              }
              n254 = for {
                N: "Soften points" -> [_]
                tunnel: w498 -> [w536]
                tunnel: [w537] -> w505 mode=concatenating
                shift-right: [w534] -> _
                shift-left: w506 -> [w538]
                tunnel: [w531] -> _ mode=indexing
                i -> [w532]
                n255 = Add(x=w532, y=1.0) -> (x+y=w531:dbl)
                n256 = Divide(x=w536, y=w531) -> (x/y=w533:dbl)
                n257 = Add(x=w538, y=w533) -> (x+y=w534:dbl)
                n258 = Build Array(w534) -> (w537:dbl[])
              }
              n259 = Multiply(x="Soften points", y=2.0) -> (x*y=w482:dbl)
              n260 = Reverse 1D Array(array=w500) -> (reversed array=w480:dbl[])
              n261 = Reverse 1D Array(array=w505) -> (reversed array=w481:dbl[])
              n262 = Build Array (concatenate)(w500, w480) -> (w497:dbl[])
              n263 = Build Array (concatenate)(w505, w481) -> (w503:dbl[])
              n264 = Add(x=w482, y=w479) -> (x+y=w493:dbl)
              n265 = call-poly <vilib>:"Ramp Pattern.vi"("type"=w514, "exclude end?"=FALSE, "start"=w507, "end"=w508, "samples"=w478) -> ("Ramp Pattern"=w473:dbl[])  [unwired: 5 in, 1 out]
              n266 = call-poly <vilib>:"Ramp Pattern.vi"("type"=w516, "exclude end?"=FALSE, "start"=w499, "end"=w506, "samples"=w479) -> ("Ramp Pattern"=w504:dbl[])  [unwired: 5 in, 1 out]
              n267 = Multiply(x=w493, y=w478) -> (x*y=w489:dbl)
              n268 = Reverse 1D Array(array=w504) -> (reversed array=w502:dbl[])
              n269 = Build Array (concatenate)(w504, w502) -> ()  [unwired: 1 out]
              n270 = Build Array (concatenate)(w504, w503, w502, w497) -> (w496:dbl[])
              n271 = Reverse 1D Array(array=w473) -> (reversed array=w512:dbl[])
              n272 = for {
                N: w478 -> [_]
                tunnel: w473 -> [w543] mode=indexing
                tunnel: [w539] -> w474 mode=concatenating
                tunnel: w482 -> [w540]
                n273 = local read "Fast-axis Para"() -> (w546:T2)
                n274 = Unbundle By Name(w546) -> ("Number of Steps"=w541:i32)
                n275 = Add(x=w540, y=w541) -> (x+y=w542:dbl)
                n276 = Multiply(x=w542, y=2) -> (x*y=w544:dbl)
                n277 = Initialize Array(w543, w544) -> (w539:dbl[])
              }
              n278 = Max & Min(x=w478, y=w479) -> (max(x,y)=w522:i32)  [unwired: 1 out]
              n279 = Multiply(x=w478, y=w479) -> (x*y=w477:i32)
              n280 = case shown="False" w510 {
                tunnel: w512 -> [w547 _]
                tunnel: [w547 dbl[] []] -> w511
                frame True {
                }
                frame False {
                }
              }
              n281 = Divide(x=w477, y=w522) -> (x/y=w491:dbl)
              n282 = Round Toward -Infinity(1:w491) -> (0:w492:dbl)
              n283 = Multiply(x=2.0, y=w489) -> (x*y=w517:dbl)
              n284 = local read "Fast-axis Para"() -> (w521:T2)
              n285 = Unbundle By Name(w521) -> ("Number of Steps"=w495:i32, "Min X"=w487:dbl)  [unwired: 1 out]
              n286 = case shown="True" w510 {
                tunnel: [w553 w556] -> w485
                tunnel: w492 -> [w549 _]
                tunnel: w517 -> [w555 w559]
                tunnel: w487 -> [w554 w558]
                tunnel: [w550 w557] -> w484
                frame True {
                  n287 = Add(x=w555, y=w549) -> (x+y=w551:dbl)
                  n288 = Initialize Array(w554, w551) -> (w553:dbl[])
                  n289 = Array Size(array=w553) -> (size(s)=w552:i32)
                  n290 = Subtract(x=w552, y=w549) -> (x-y=w550:dbl)
                }
                frame False {
                  n291 = Initialize Array(w558, w559) -> (w556:dbl[])
                  n292 = Array Size(array=w556) -> (size(s)=w557:i32)
                }
              }
              n293 = local read "Slow-axis Para"() -> (w520:T1)
              n294 = Unbundle By Name(w520) -> ("Number of Steps"=w490:i32)  [unwired: 2 out]
              n295 = Add(x=w495, y=w482) -> (x+y=w494:dbl)
              n296 = for {
                N: w490 -> [_]
                tunnel: w496 -> [w567]
                shift-right: [w560] -> w476
                shift-left: w485 -> [w566]
                tunnel: w494 -> [w565]
                i -> [w561]
                n297 = Multiply(x=w561, y=w565) -> (x*y=w563:dbl)
                n298 = Multiply(x=2.0, y=w563) -> (x*y=w562:dbl)
                n299 = Replace Array Subset(array=w566, new element=w567, index=w562) -> (w560:dbl[])
              }
              n300 = Build Array (concatenate)(w474, w511) -> (w519:dbl[])
              n301 = Subtract(x=w484, y=w482) -> (x-y=w488:dbl)
              n302 = Initialize Array(w487, w482) -> (w486:dbl[])
              n303 = Replace Array Subset(array=w476, new element=w486, index=w488) -> ()  [unwired: 1 out]
              n304 = Build Array(w519, w476) -> (w509:dbl[][])
            }
            frame False {
              w587 = u16 0 items=["Linear", "Logarithmic"] ("type")
              w589 = u16 0 items=["Linear", "Logarithmic"] ("type")
              n305 = Multiply(x=w572, y=w579) -> (x*y=w581:i32)
              n306 = call-poly <vilib>:"Ramp Pattern.vi"("type"=w587, "exclude end?"=FALSE, "start"=w575, "end"=w576, "samples"=w579) -> ("Ramp Pattern"=w584:dbl[])  [unwired: 5 in, 1 out]
              n307 = call-poly <vilib>:"Ramp Pattern.vi"("type"=w589, "exclude end?"=FALSE, "start"=w570, "end"=w571, "samples"=w572) -> ("Ramp Pattern"=w574:dbl[])  [unwired: 5 in, 1 out]
              n308 = Reverse 1D Array(array=w574) -> (reversed array=w573:dbl[])
              n309 = Build Array (concatenate)(w574, w573) -> (w568:dbl[])
              n310 = Reverse 1D Array(array=w584) -> (reversed array=w583:dbl[])
              n311 = for {
                N: w579 -> [_]
                tunnel: w584 -> [w602] mode=indexing
                tunnel: [w601] -> w585 mode=concatenating
                n312 = local read "Fast-axis Para"() -> (w606:T2)
                n313 = Unbundle By Name(w606) -> ("Number of Steps"=w605:i32)
                n314 = Multiply(x=w605, y=2) -> (x*y=w603:i32)
                n315 = Initialize Array(w602, w603) -> (w601:dbl[])
              }
              n316 = Max & Min(x=w572, y=w572) -> (max(x,y)=w599:i32)  [unwired: 1 out]
              n317 = case shown="True" w578 {
                tunnel: w583 -> [w607 _]
                tunnel: [w607 dbl[] []] -> w582
                frame True {
                }
                frame False {
                }
              }
              n318 = Divide(x=w581, y=w599) -> (x/y=w598:dbl)
              n319 = Multiply(x=2.0, y=w581) -> (x*y=w590:dbl)
              n320 = local read "Fast-axis Para"() -> (w597:T2)
              n321 = Unbundle By Name(w597) -> ("Number of Steps"=w596:i32, "Min X"=w569:dbl)  [unwired: 1 out]
              n322 = case shown="True" w578 {
                tunnel: [w613 w615] -> w600
                tunnel: w598 -> [w612 _]
                tunnel: w590 -> [w610 w614]
                tunnel: w569 -> [w609 _]
                frame True {
                  n323 = Add(x=w610, y=w612) -> (x+y=w611:dbl)
                  n324 = Initialize Array(w609, w611) -> (w613:dbl[])
                }
                frame False {
                  n325 = Initialize Array(0.0 ("element"), w614) -> (w615:dbl[])
                }
              }
              n326 = local read "Slow-axis Para"() -> (w595:T1)
              n327 = Unbundle By Name(w595) -> ("Number of Steps"=w593:i32)  [unwired: 2 out]
              n328 = Increment(x=w593) -> (x+1=w592:i32)
              n329 = for {
                N: w592 -> [_]
                tunnel: w568 -> [w625]
                shift-right: [w623] -> w580
                shift-left: w600 -> [w624]
                tunnel: w596 -> [w622]
                i -> [w621]
                n330 = Decrement(x=w621) -> (x-1=w620:i32)
                n331 = Multiply(x=w620, y=w622) -> (x*y=w618:i32)
                n332 = Multiply(x=2.0, y=w618) -> (x*y=w617:dbl)
                n333 = Replace Array Subset(array=w624, new element=w625, index=w617) -> (w623:dbl[])
              }
              n334 = Build Array (concatenate)(w585, w582) -> (w594:dbl[])
              n335 = Build Array(w594, w580) -> (w577:dbl[][])
            }
          }
        }
        frame "Bi-Directional" {
          n336 = local read "Soften"() -> (w626:bool)
          n337 = case shown="True" w626 {
            tunnel: w634 -> [w645 w774]
            tunnel: w633 -> [w683 w773]
            tunnel: w632 -> [w656 w772]
            tunnel: w631 -> [w655 w771]
            tunnel: w630 -> [w682 w770]
            tunnel: w629 -> [w681 w769]
            tunnel: [w677 w765] -> w628
            tunnel: w627 -> [w650 w750]
            frame True {
              w690 = u16 0 items=["Linear", "Logarithmic"] ("type")
              w692 = u16 0 items=["Linear", "Logarithmic"] ("type")
              n338 = Decrement(x=w645) -> (x-1=w662:i32)
              n339 = Divide(x=w656, y=w662) -> (x/y=w660:dbl)
              n340 = local read "Soften points"() -> (w657:i32)
              n341 = for {
                N: w657 -> [_]
                tunnel: w660 -> [w706]
                tunnel: [w707] -> w661 mode=concatenating
                shift-right: [w704] -> _
                shift-left: w655 -> [w708]
                tunnel: [w701] -> _ mode=indexing
                i -> [w702]
                n342 = Add(x=w702, y=1.0) -> (x+y=w701:dbl)
                n343 = Divide(x=w706, y=w701) -> (x/y=w703:dbl)
                n344 = Subtract(x=w708, y=w703) -> (x-y=w704:dbl)
                n345 = Build Array(w704) -> (w707:dbl[])
              }
              n346 = for {
                N: w657 -> [_]
                tunnel: w660 -> [w714]
                tunnel: [w715] -> w663 mode=concatenating
                shift-right: [w712] -> _
                shift-left: w656 -> [w716]
                tunnel: [w709] -> _ mode=indexing
                i -> [w710]
                n347 = Add(x=w710, y=1.0) -> (x+y=w709:dbl)
                n348 = Divide(x=w714, y=w709) -> (x/y=w711:dbl)
                n349 = Add(x=w716, y=w711) -> (x+y=w712:dbl)
                n350 = Build Array(w712) -> (w715:dbl[])
              }
              n351 = Quotient & Remainder(x=w650, y=2.0) -> (x-y*floor(x/y)=w673:dbl)  [unwired: 1 out]
              n352 = Equal To 0?(x=w673) -> (x = 0?=w672:bool)
              n353 = Reverse 1D Array(array=w661) -> (reversed array=w658:dbl[])
              n354 = Reverse 1D Array(array=w663) -> (reversed array=w659:dbl[])
              n355 = local read "Soften points"() -> (w647:i32)
              n356 = case shown="True" w672 {
                tunnel: w650 -> [w718 w719]
                tunnel: [w717 w719] -> w671
                frame False {
                  n357 = Increment(x=w718) -> (x+1=w717:i32)
                }
                frame True {
                }
              }
              n358 = Build Array (concatenate)(w661, w658) -> (w651:dbl[])
              n359 = Build Array (concatenate)(w663, w659) -> (w653:dbl[])
              n360 = Multiply(x=w647, y=2.0) -> (x*y=w646:dbl)
              n361 = Add(x=w646, y=w645) -> (x+y=w644:dbl)
              n362 = Multiply(x=w644, y=w671) -> (x*y=w684:dbl)
              n363 = call-poly <vilib>:"Ramp Pattern.vi"("type"=w690, "exclude end?"=FALSE, "start"=w681, "end"=w682, "samples"=w650) -> ("Ramp Pattern"=w687:dbl[])  [unwired: 5 in, 1 out]
              n364 = call-poly <vilib>:"Ramp Pattern.vi"("type"=w692, "exclude end?"=FALSE, "start"=w655, "end"=w656, "samples"=w645) -> ("Ramp Pattern"=w654:dbl[])  [unwired: 5 in, 1 out]
              n365 = Reverse 1D Array(array=w654) -> (reversed array=w652:dbl[])
              n366 = Build Array (concatenate)(w654, w652) -> ()  [unwired: 1 out]
              n367 = Reverse 1D Array(array=w687) -> (reversed array=w686:dbl[])
              n368 = Max & Min(x=w645, y=w650) -> (max(x,y)=w699:i32)  [unwired: 1 out]
              n369 = Build Array (concatenate)(w654, w653, w652, w651) -> (w641:dbl[])
              n370 = Multiply(x=w645, y=w650) -> (x*y=w649:i32)
              n371 = case shown="False" w683 {
                tunnel: w686 -> [w726 _]
                tunnel: [w726 dbl[] []] -> w685
                frame True {
                }
                frame False {
                }
              }
              n372 = Divide(x=w649, y=w699) -> (x/y=w698:dbl)
              n373 = Multiply(x=1.0, y=w684) -> (x*y=w693:dbl)
              n374 = local read "Fast-axis Para"() -> (w697:T2)
              n375 = Unbundle By Name(w697) -> ("Number of Steps"=w696:i32, "Min X"=w639:dbl)  [unwired: 1 out]
              n376 = case shown="False" w683 {
                tunnel: [w731 w736] -> w700
                tunnel: w698 -> [w734 _]
                tunnel: w693 -> [w733 w737]
                tunnel: w639 -> [w732 _]
                tunnel: [w728 w735] -> w636
                frame True {
                  n377 = Add(x=w733, y=w734) -> (x+y=w729:dbl)
                  n378 = Initialize Array(w732, w729) -> (w731:dbl[])
                  n379 = Array Size(array=w731) -> (size(s)=w730:i32)
                  n380 = Subtract(x=w730, y=w729) -> (x-y=w728:dbl)
                }
                frame False {
                  n381 = Initialize Array(0.0 ("element"), w737) -> (w736:dbl[])
                  n382 = Array Size(array=w736) -> (size(s)=w735:i32)
                }
              }
              n383 = local read "Slow-axis Para"() -> (w695:T1)
              n384 = local read "Soften points"() -> (w642:i32)
              n385 = Unbundle By Name(w695) -> ("Number of Steps"=w679:i32, "Min Y"=w667:dbl)  [unwired: 1 out]
              n386 = Divide(x=w679, y=2.0) -> (x/y=w678:dbl)
              n387 = Multiply(x=w642, y=2.0) -> (x*y=w637:dbl)
              n388 = for {
                N: w650 -> [_]
                tunnel: w687 -> [w722] mode=indexing
                tunnel: [w721] -> w688 mode=concatenating
                tunnel: w637 -> [w720]
                n389 = local read "Fast-axis Para"() -> (w725:T2)
                n390 = Unbundle By Name(w725) -> ("Number of Steps"=w724:i32)
                n391 = Add(x=w724, y=w720) -> (x+y=w723:dbl)
                n392 = Initialize Array(w722, w723) -> (w721:dbl[])
              }
              n393 = Increment(x=w678) -> (x+1=w676:dbl)
              n394 = Round Toward +Infinity(x=w676) -> (ceil(x): smallest int >= x=w675:dbl)
              n395 = for {
                N: w675 -> [_]
                tunnel: w641 -> [w749]
                shift-right: [w747] -> w635
                shift-left: w700 -> [w748]
                tunnel: w696 -> [w740]
                tunnel: w637 -> [w741]
                i -> [w746]
                n396 = Decrement(x=w746) -> (x-1=w745:i32)
                n397 = Add(x=w740, y=w741) -> (x+y=w739:dbl)
                n398 = Multiply(x=w745, y=w739) -> (x*y=w743:dbl)
                n399 = Multiply(x=2.0, y=w743) -> (x*y=w742:dbl)
                n400 = Replace Array Subset(array=w748, new element=w749, index=w742) -> (w747:dbl[])
              }
              n401 = Build Array (concatenate)(w688, w685) -> (w666:dbl[])
              n402 = Array Size(array=w666) -> (size(s)=w669:i32)
              n403 = Array Size(array=w635) -> (size(s)=w670:i32)
              n404 = Subtract(x=w670, y=w669) -> (x-y=w668:i32)
              n405 = Subtract(x=w636, y=w637) -> (x-y=w640:dbl)
              n406 = Initialize Array(w639, w637) -> (w638:dbl[])
              n407 = Initialize Array(w667, w668) -> (w665:dbl[])
              n408 = Replace Array Subset(array=w635, new element=w638, index=w640) -> ()  [unwired: 1 out]
              n409 = Build Array (concatenate)(w666, w665) -> (w664:dbl[])
              n410 = Build Array(w664, w635) -> (w677:dbl[][])
            }
            frame False {
              w783 = u16 0 items=["Linear", "Logarithmic"] ("type")
              w787 = u16 0 items=["Linear", "Logarithmic"] ("type")
              n411 = Quotient & Remainder(x=w750, y=2.0) -> (x-y*floor(x/y)=w761:dbl)  [unwired: 1 out]
              n412 = Equal To 0?(x=w761) -> (x = 0?=w760:bool)
              n413 = case shown="False" w760 {
                tunnel: w750 -> [w797 w798]
                tunnel: [w796 w798] -> w759
                frame False {
                  n414 = Increment(x=w797) -> (x+1=w796:i32)
                }
                frame True {
                }
              }
              n415 = Multiply(x=w774, y=w759) -> (x*y=w776:i32)
              n416 = call-poly <vilib>:"Ramp Pattern.vi"("type"=w783, "exclude end?"=FALSE, "start"=w769, "end"=w770, "samples"=w750) -> ("Ramp Pattern"=w780:dbl[])  [unwired: 5 in, 1 out]
              n417 = call-poly <vilib>:"Ramp Pattern.vi"("type"=w787, "exclude end?"=FALSE, "start"=w771, "end"=w772, "samples"=w774) -> ("Ramp Pattern"=w784:dbl[])  [unwired: 5 in, 1 out]
              n418 = Reverse 1D Array(array=w784) -> (reversed array=w777:dbl[])
              n419 = Build Array (concatenate)(w784, w777) -> (w785:dbl[])
              n420 = Reverse 1D Array(array=w780) -> (reversed array=w779:dbl[])
              n421 = for {
                N: w750 -> [_]
                tunnel: w780 -> [w800] mode=indexing
                tunnel: [w799] -> w781 mode=concatenating
                n422 = local read "Fast-axis Para"() -> (w804:T2)
                n423 = Unbundle By Name(w804) -> ("Number of Steps"=w803:i32)
                n424 = Multiply(x=w803, y=1) -> (x*y=w801:i32)
                n425 = Initialize Array(w800, w801) -> (w799:dbl[])
              }
              n426 = Max & Min(x=w774, y=w750) -> (max(x,y)=w794:i32)  [unwired: 1 out]
              n427 = case shown="False" w773 {
                tunnel: w779 -> [w805 _]
                tunnel: [w805 dbl[] []] -> w778
                frame True {
                }
                frame False {
                }
              }
              n428 = Divide(x=w776, y=w794) -> (x/y=w793:dbl)
              n429 = Multiply(x=1.0, y=w776) -> (x*y=w788:dbl)
              n430 = local read "Fast-axis Para"() -> (w792:T2)
              n431 = Unbundle By Name(w792) -> ("Number of Steps"=w791:i32, "Min X"=w775:dbl)  [unwired: 1 out]
              n432 = case shown="False" w773 {
                tunnel: [w811 w813] -> w795
                tunnel: w793 -> [w810 _]
                tunnel: w788 -> [w808 w812]
                tunnel: w775 -> [w807 _]
                frame True {
                  n433 = Add(x=w808, y=w810) -> (x+y=w809:dbl)
                  n434 = Initialize Array(w807, w809) -> (w811:dbl[])
                }
                frame False {
                  n435 = Initialize Array(0.0 ("element"), w812) -> (w813:dbl[])
                }
              }
              n436 = local read "Slow-axis Para"() -> (w790:T1)
              n437 = Unbundle By Name(w790) -> ("Number of Steps"=w767:i32, "Min Y"=w754:dbl)  [unwired: 1 out]
              n438 = Divide(x=w767, y=2.0) -> (x/y=w766:dbl)
              n439 = Increment(x=w766) -> (x+1=w764:dbl)
              n440 = Round Toward +Infinity(x=w764) -> (ceil(x): smallest int >= x=w763:dbl)
              n441 = for {
                N: w763 -> [_]
                tunnel: w785 -> [w823]
                shift-right: [w821] -> w758
                shift-left: w795 -> [w822]
                tunnel: w791 -> [w820]
                i -> [w819]
                n442 = Decrement(x=w819) -> (x-1=w818:i32)
                n443 = Multiply(x=w818, y=w820) -> (x*y=w816:i32)
                n444 = Multiply(x=2.0, y=w816) -> (x*y=w815:dbl)
                n445 = Replace Array Subset(array=w822, new element=w823, index=w815) -> (w821:dbl[])
              }
              n446 = Build Array (concatenate)(w781, w778) -> (w753:dbl[])
              n447 = Array Size(array=w753) -> (size(s)=w756:i32)
              n448 = Array Size(array=w758) -> (size(s)=w757:i32)
              n449 = Subtract(x=w757, y=w756) -> (x-y=w755:i32)
              n450 = Initialize Array(w754, w755) -> (w752:dbl[])
              n451 = Build Array (concatenate)(w753, w752) -> (w751:dbl[])
              n452 = Build Array(w751, w758) -> (w765:dbl[][])
            }
          }
        }
      }
    }
    frame Error {
    }
  }
  "error IO" <- w21
  n453 = local read "Reset slow axis at End of Scan?"() -> (w5:bool)
  n454 = local read "Slow-axis Para"() -> (w10:T1)
  n455 = Index Array(array=w24, index (row)=1) -> (element=w15:dbl[])  [unwired: 1 in]
  n456 = Index Array(array=w24, index (row)=u8 0) -> (element=w13:dbl[])  [unwired: 1 in]
  n457 = local read "Fast-axis Para"() -> (w7:T2)
  n458 = case shown="False" w5 {
    tunnel: w10 -> [w827 w829]
    tunnel: [w826 w828] -> w2
    frame True {
      n459 = Unbundle By Name(w827) -> ("Min Y"=w826:dbl)
    }
    frame False {
      n460 = Unbundle By Name(w829) -> ("Max Y"=w828:dbl)
    }
  }
  n461 = Unbundle By Name(w7) -> ("Min X"=w4:dbl)
  n462 = local read "Pattern"() -> (w23:T3)
  n463 = Equal?(x=w23, y=T3."Lissajous") -> (x = y?=w18:bool)
  n464 = case shown="False" w18 {
    tunnel: w2 -> [w830 _]
    tunnel: [w830 0.0 ("Max Y")] -> w1
    frame False {
    }
    frame True {
    }
  }
  n465 = case shown="False" w18 {
    tunnel: w4 -> [w832 _]
    tunnel: [w832 0.0 ("Min X")] -> w3
    frame False {
    }
    frame True {
    }
  }
  n466 = Initialize Array(w1, 100 ("dimension size")) -> (w9:dbl[])
  n467 = Initialize Array(w3, 100 ("dimension size")) -> (w6:dbl[])
  n468 = Build Array (concatenate)(w15, w6) -> (w14:dbl[])
  n469 = Build Array (concatenate)(w13, w9) -> (w12:dbl[])
  n470 = Build Array(w14, w12) -> (→"2D Raster Pattern":dbl[][])
